vi "MH_CalcDeltaTNegB.vi"(0 "Buffindex":i32, 1 "TrueTime":u64, 3 "Buffsize":i32, 5 "Data In":u64[](array[numeric]), 7 "DeltasBuffer":i32[](array[numeric]), 9 "Deltaindex":i32, 11 "DBuffSize":i32=10, 12 "WinIndex":i32, 13 "WIndowW":i32) -> (4 "Write Delta":bool, 6 "NewDelta":bool, 8 "DeltasBufferOut":i32[](array[numeric]), 10 "DeltaIndexOut":i32, 14 "WinIndexOut":i32, 15 "DBuffSize out":i32=10)   [LabVIEW 2019]
uses:
  <userlib>/MultiHarp150/T2Lib/MH_T2DeltaQMessage.ctl
panel:
  in  "queue out":refnum<queue>
  # "here"
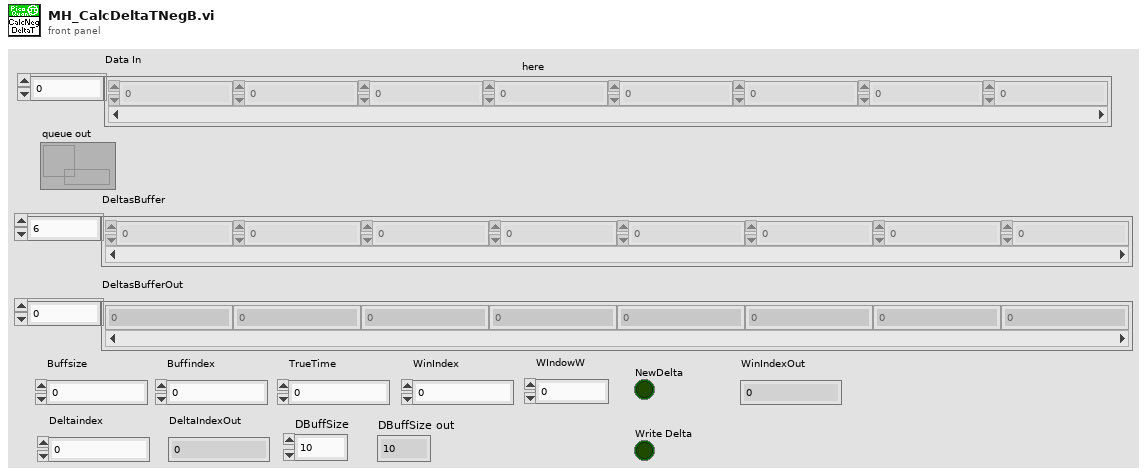
[diagram p1: front panel]
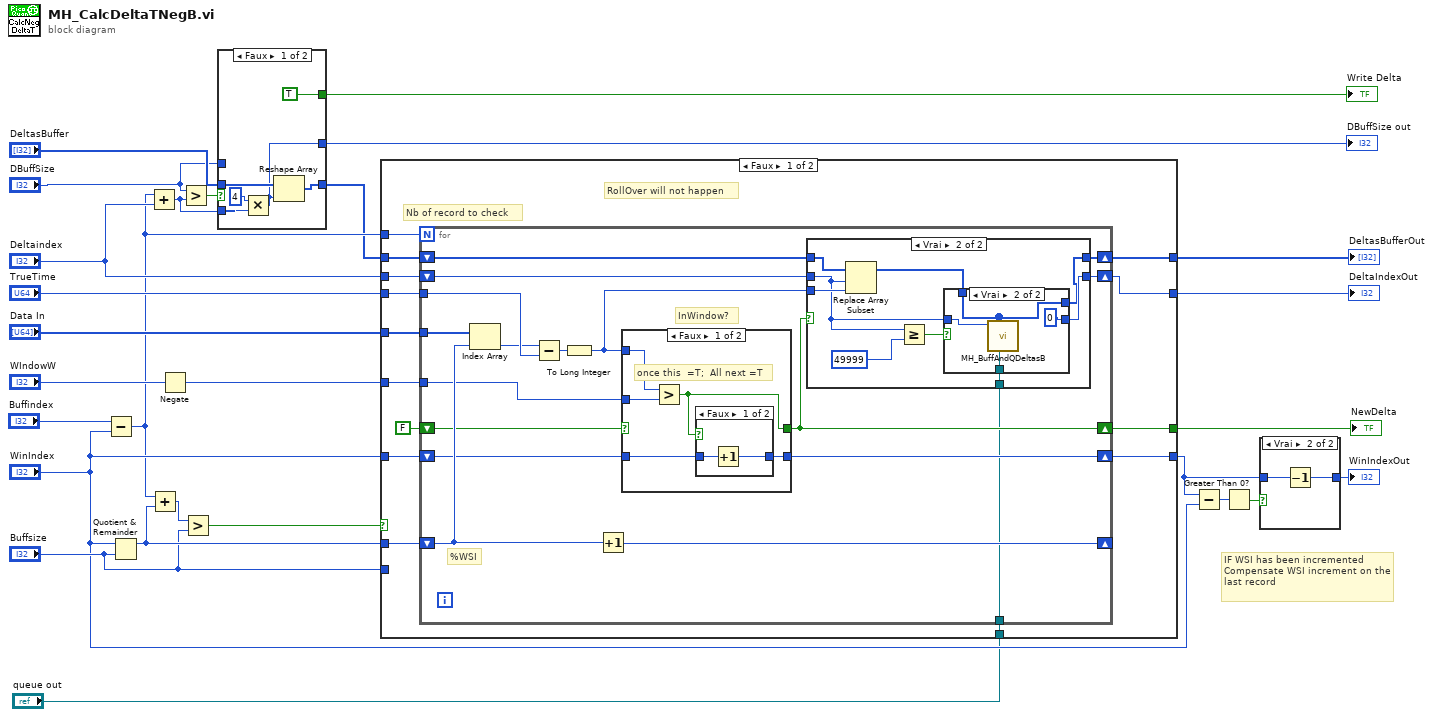
[diagram p0: block diagram]
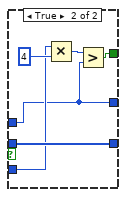
[diagram p2: hidden frame]
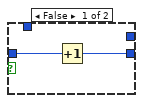
[diagram p4: hidden frame]
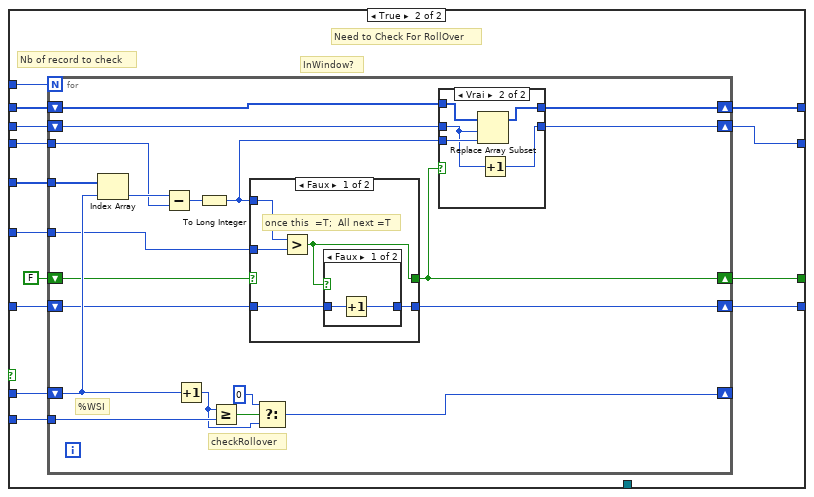
[diagram p7: hidden frame]
diagram:
  # "IF WSI has been incremented\nCompensate WSI increment on the last record"
  n1 = Subtract(x="Buffindex", y="WinIndex") -> (x-y=w9:i32)
  n2 = Quotient & Remainder(x="WinIndex", y="Buffsize") -> (x-y*floor(x/y)=w18:i32)  [unwired: 1 out]
  n3 = Add(x=w9, y="Deltaindex") -> (x+y=w5:i32)
  n4 = Add(x=w9, y=w18) -> (x+y=w17:i32)
  n5 = Negate(x="WIndowW") -> (-x=w14:i32)
  n6 = Greater?(x="DBuffSize", y=w5) -> (0:w8:bool)
  n7 = Greater?(x=w17, y="Buffsize") -> (0:w15:bool)
  n8 = case shown="Faux" w8 {
    tunnel: [w32 w39] -> w6
    tunnel: "DeltasBuffer" -> [w33 w39]
    tunnel: w5 -> [w31 w36]
    tunnel: [w29 w34] -> w4
    tunnel: "DBuffSize" -> [_ w34]
    tunnel: [TRUE w35] -> w2
    frame False {
      n9 = Multiply(x=4, y=w31) -> (x*y=w29:i32)
      n10 = Reshape Array(w33, w29) -> (w32:i32[])
    }
    frame True {
      n11 = Multiply(x=w36, y=4) -> (x*y=w38:i32)
      n12 = Greater?(x=w38, y=w34) -> (0:w35:bool)
    }
  }
  "DBuffSize out" <- w4
  "Write Delta" <- w2
  n13 = case shown="Faux" w15 {
    tunnel: "Data In" -> [w53 w111]
    tunnel: "TrueTime" -> [w52 w110]
    tunnel: w14 -> [w51 w109]
    tunnel: [w50 w108] -> w23
    tunnel: "WinIndex" -> [w48 w106]
    tunnel: [w47 w105] -> w19
    tunnel: w9 -> [w46 w104]
    tunnel: w18 -> [w45 w103]
    tunnel: "Buffsize" -> [_ w102]
    tunnel: w6 -> [w44 w101]
    tunnel: "Deltaindex" -> [w43 w100]
    tunnel: [w42 w99] -> w13
    tunnel: [w41 w98] -> w12
    tunnel: "queue out" -> [w40 _]
    frame False {
      # "RollOver will not happen"
      # "Nb of record to check"
      n14 = for {
        N: w46 -> [_]
        tunnel: w53 -> [w70]
        tunnel: w52 -> [w62]
        shift-right: [w64] -> w47
        shift-left: w48 -> [w65]
        shift-right: [w63] -> _
        shift-left: w45 -> [w68]
        tunnel: w51 -> [w67]
        shift-right: [w55] -> w50
        shift-left: FALSE -> [w66]
        shift-right: [w56] -> w42
        shift-left: w44 -> [w60]
        shift-right: [w57] -> w41
        shift-left: w43 -> [w58]
        tunnel: w40 -> [w54]
        # "InWindow?"
        # "%WSI"
        n15 = Index Array(array=w70, index=w68) -> (element=w61:u64)
        n16 = Subtract(x=w61, y=w62) -> (x-y=w69:u64)
        n17 = To Long Integer(number=w69) -> (32bit integer=w59:i32)
        n18 = Increment(x=w68) -> (x+1=w63:i32)
        n19 = case shown="Faux" w66 {
          selector: w66 -> [_ w96]
          tunnel: w59 -> [w92 _]
          tunnel: w67 -> [w91 _]
          tunnel: [w88 w96] -> w55
          tunnel: w65 -> [w90 w97]
          tunnel: [w89 w97] -> w64
          frame False {
            # "once this  =T;  All next =T"
            n20 = Greater?(x=w92, y=w91) -> (0:w88:bool)
            n21 = case shown="Faux" w88 {
              tunnel: w90 -> [w94 w95]
              tunnel: [w93 w95] -> w89
              frame False {
                n22 = Increment(x=w94) -> (x+1=w93:i32)
              }
              frame True {
              }
            }
          }
          frame True {
          }
        }
        n23 = case shown="Vrai" w55 {
          tunnel: w60 -> [w72 w80]
          tunnel: w59 -> [_ w81]
          tunnel: w58 -> [w71 w76]
          tunnel: [w71 w75] -> w57
          tunnel: [w72 w73] -> w56
          tunnel: w54 -> [_ w74]
          frame False {
          }
          frame True {
            n24 = Replace Array Subset(array=w80, new element=w81, index=w76) -> (w77:i32[])
            n25 = Greater Or Equal?(x=w76, y=49999) -> (x >= y?=w78:bool)
            n26 = case shown="Vrai" w78 {
              tunnel: w77 -> [_ w84]
              tunnel: w76 -> [w83 w85]
              tunnel: [w82 0] -> w75
              tunnel: w74 -> [_ w87]
              tunnel: [_ w84] -> w73
              frame False {
                n27 = Increment(x=w83) -> (x+1=w82:i32)
              }
              frame True {
                n28 = call <userlib>:"MH_BuffAndQDeltasB.vi"("queue out"=w87, "DeltasBuffer"=w84, "DBuffSize"=w85) -> ()  [unwired: 8 in, 1 out]
              }
            }
          }
        }
      }
    }
    frame True {
      # "InWindow?"
      # "Need to Check For RollOver"
      # "Nb of record to check"
      n29 = for {
        N: w104 -> [_]
        tunnel: w111 -> [w131]
        tunnel: w110 -> [w119]
        shift-right: [w124] -> w105
        shift-left: w106 -> [w125]
        shift-right: [w128] -> _
        shift-left: w103 -> [w129]
        tunnel: w102 -> [w130]
        tunnel: w109 -> [w127]
        shift-right: [w112] -> w108
        shift-left: FALSE -> [w126]
        shift-right: [w117] -> w99
        shift-left: w101 -> [w115]
        shift-right: [w116] -> w98
        shift-left: w100 -> [w114]
        # "checkRollover"
        # "%WSI"
        n30 = Index Array(array=w131, index=w129) -> (element=w120:u64)
        n31 = Subtract(x=w120, y=w119) -> (x-y=w118:u64)
        n32 = Increment(x=w129) -> (x+1=w121:i32)
        n33 = To Long Integer(number=w118) -> (32bit integer=w113:i32)
        n34 = Greater Or Equal?(x=w121, y=w130) -> (x >= y?=w123:bool)
        n35 = case shown="Faux" w126 {
          selector: w126 -> [_ w147]
          tunnel: w113 -> [w143 _]
          tunnel: w127 -> [w142 _]
          tunnel: [w139 w147] -> w112
          tunnel: w125 -> [w141 w148]
          tunnel: [w140 w148] -> w124
          frame False {
            # "once this  =T;  All next =T"
            n36 = Greater?(x=w143, y=w142) -> (0:w139:bool)
            n37 = case shown="Faux" w139 {
              tunnel: w141 -> [w145 w146]
              tunnel: [w144 w146] -> w140
              frame False {
                n38 = Increment(x=w145) -> (x+1=w144:i32)
              }
              frame True {
              }
            }
          }
          frame True {
          }
        }
        n39 = Select(t=0 ("x+1"), s=w123, f=w121) -> (s? t:f=w128:i32)
        n40 = case shown="Vrai" w112 {
          tunnel: w115 -> [w133 w135]
          tunnel: w113 -> [_ w138]
          tunnel: w114 -> [w132 w134]
          tunnel: [w132 w137] -> w116
          tunnel: [w133 w136] -> w117
          frame False {
          }
          frame True {
            n41 = Replace Array Subset(array=w135, new element=w138, index=w134) -> (w136:i32[])
            n42 = Increment(x=w134) -> (x+1=w137:i32)
          }
        }
      }
    }
  }
  "NewDelta" <- w23
  "DeltasBufferOut" <- w13
  "DeltaIndexOut" <- w12
  n43 = Subtract(x=w19, y="WinIndex") -> (x-y=w22:i32)
  n44 = Greater Than 0?(x=w22) -> (x > 0?=w21:bool)
  n45 = case shown="Vrai" w21 {
    tunnel: [w149 w150] -> w20
    tunnel: w19 -> [w149 w151]
    frame False {
    }
    frame True {
      n46 = Decrement(x=w151) -> (x-1=w150:i32)
    }
  }
  "WinIndexOut" <- w20
